vi "Stop ExampleDependency.vi"(8 "error in (no error)":errorcluster, 10 "Dependency Name":string, 11 "SMO.Example in":refnum<class "SMO.Example.lvclass">) -> (0 "error out":errorcluster, 3 "SMO.Example out":refnum<class "SMO.Example.lvclass">)   [LabVIEW 2013, in "SMO.Example.lvclass"]
uses:
  SMO.Example.lvclass
  SMO/SMO.lvclass
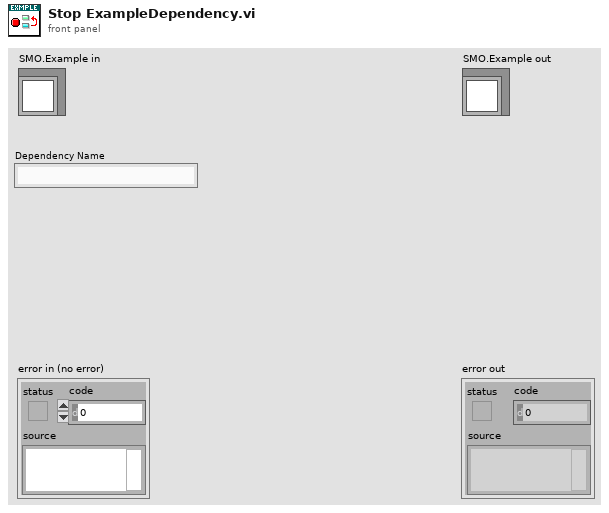
[diagram p1: front panel]
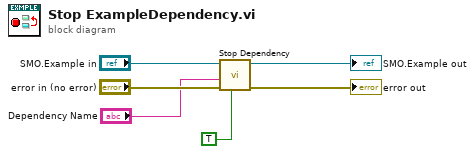
[diagram p0: block diagram]
diagram:
  n1 = call "Stop Dependency.vi"("Destroy ref? (T)"=TRUE, "error in (no error)"="error in (no error)", "Name (ignored if reference valid)"="Dependency Name", "SMO in"="SMO.Example in") -> ("error out"=→"error out":errorcluster, "SMO out"=→"SMO.Example out":refnum<class "SMO.Example.lvclass">)  [unwired: 5 in, 1 out]
